vi "Single Clothoid Calculation.vi"(9 "Angle":dbl, 10 "Min R":dbl) -> (3 "Zeroes out":T1)   [LabVIEW 2018]
uses:
  BlendType.ctl
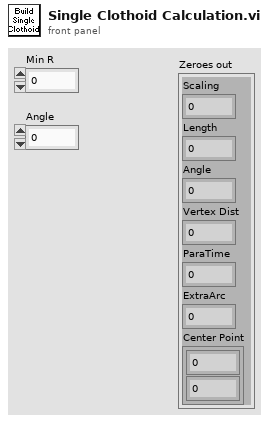
[diagram p1: front panel]
types:
  T1 = typedef "BlendType.ctl" = cluster{"Scaling":dbl, "Length":dbl, "Angle":dbl, "Vertex Dist":dbl, "ParaTime":dbl, "ExtraArc":dbl, "Center Point":cluster{dbl, dbl}}
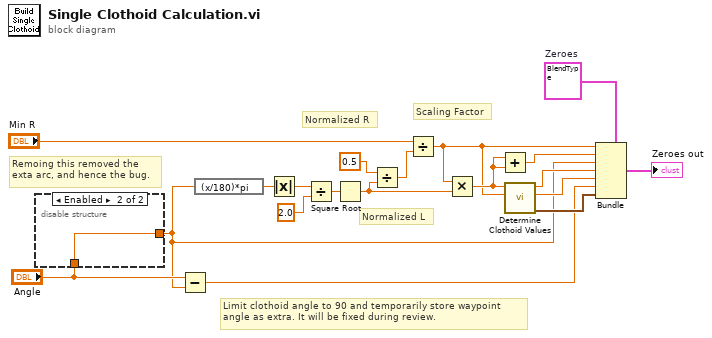
[diagram p0: block diagram]
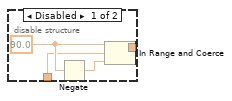
[diagram p2: hidden frame]
diagram:
  w5 = T1 {"Scaling"=0.0, "Length"=0.0, "Angle"=0.0, "Vertex Dist"=0.0, "ParaTime"=0.0, "ExtraArc"=0.0, "Center Point"={0.0, 0.0}}  # Zeroes
  # "Remoing this removed the\nexta arc, and hence the bug."
  # "Limit clothoid angle to 90 and temporarily store waypoint\nangle as extra. It will be fixed during review."
  # "Normalized L"
  # "Scaling Factor"
  # "Normalized R"
  n1 = disable-structure shown="Enabled" {
    disable-tunnel: "Angle" -> [w21 w24]
    disable-tunnel: [w20 w24] -> w3
    frame Disabled {
      w22 = 90.0
      n2 = Negate(x=w22) -> (-x=w23:dbl)
      n3 = In Range and Coerce(upper limit=w22, x=w21, lower limit=w23) -> (coerced(x)=w20:dbl)  [unwired: 1 out]
    }
    frame Enabled {
    }
  }
  n4 = Subtract(x="Angle", y=w3) -> (x-y=w1:dbl)
  n5 = expression code="(x/180)*pi" ("radians to degrees")(w3) -> (w2:dbl)
  n6 = Absolute Value(x=w2) -> (abs(x)=w13:dbl)
  n7 = Divide(x=w13, y=2.0) -> (x/y=w9:dbl)
  n8 = Square Root(x=w9) -> (sqrt(x)=w18:dbl)
  n9 = Divide(x=0.5, y=w18) -> (x/y=w7:dbl)
  n10 = Divide(x="Min R", y=w7) -> (x/y=w15:dbl)
  n11 = Multiply(x=w15, y=w18) -> (x*y=w16:dbl)
  n12 = Add(x=w16, y=w16) -> (x+y=w17:dbl)
  n13 = call "Determine Clothoid Values.vi"("Scaling"=w15, "Desired Length"=w16) -> ("Center Point"=w19:cluster{dbl, dbl}, "Para Time"=w12:dbl, "Vertex Dist ft"=w14:dbl)  [unwired: 6 in, 1 out]
  n14 = Bundle(cluster=w5, "Scaling"=w15, "Length"=w17, "Angle"=w3, "Vertex Dist"=w14, "ParaTime"=w12, "ExtraArc"=w1, "Center Point"=w19) -> (→"Zeroes out":T1)
